vi "Arm.vi"(8 "error in (no error)":errorcluster, 10 "Arm":bool, 11 "Fault-Injection Bus in":refnum<class "Fault-Injection Bus.lvclass">) -> (0 "error out":errorcluster, 3 "Fault-Injection Bus out":refnum<class "Fault-Injection Bus.lvclass">)   [LabVIEW 2021, in "Fault-Injection Bus.lvclass"]
uses:
  Fault-Injection Bus.lvclass
  Fault-Injection Bus.lvclass/Fault-Injection Bus.ctl
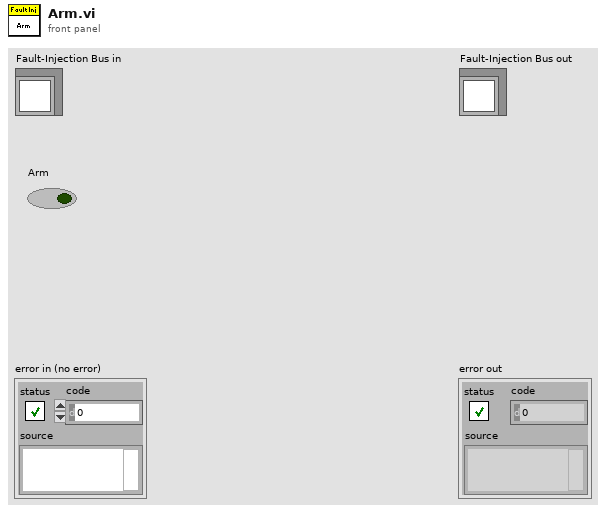
[diagram p1: front panel]
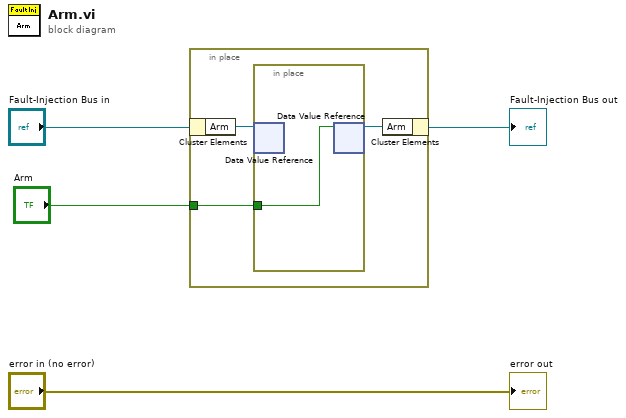
[diagram p0: block diagram]
diagram:
  n1 = in-place {
    in-place-border: "Arm" -> [w6]
    n2 = in-place-cluster #1("Fault-Injection Bus in") -> ("Arm"=w7:refnum<data-value>)
    n3 = in-place {
      in-place-border: w6 -> [w8]
      n4 = in-place-dvr #2(w7) -> ()  [unwired: 2 out]
      n5 = in-place-dvr #2(w8) -> (w5:refnum<data-value>)  [unwired: 1 out]
    }
    n6 = in-place-cluster #1("Arm"=w5) -> (→"Fault-Injection Bus out":refnum<class "Fault-Injection Bus.lvclass">)
  }
  "error out" <- "error in (no error)"
